vi "PCM_decode.vi"(8 "error in":errorcluster, 10 "inputData":dbl[](array[numeric]), 11 "Path In":path) -> (0 "error out":errorcluster, 2 "outData":dbl[](array[numeric]), 3 "Path Out":path)   [LabVIEW 2015]
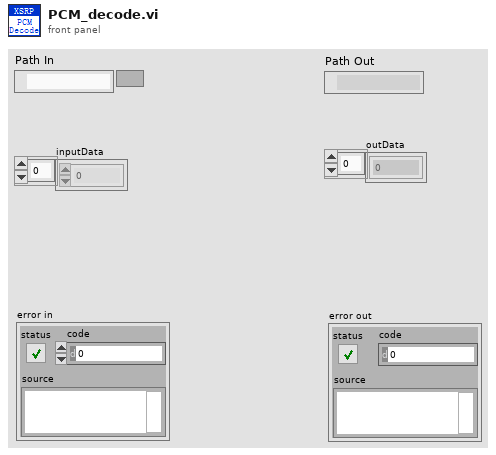
[diagram p1: front panel]
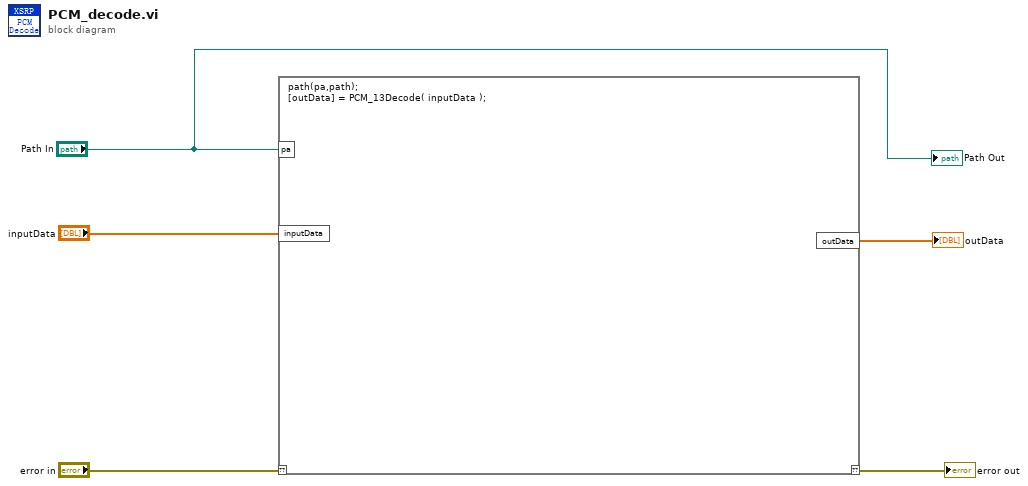
[diagram p0: block diagram]
diagram:
  n1 = script code="path(pa,path);\n[outData] = PCM_13Decode( inputData );"("??"="error in", "pa"="Path In", "inputData"="inputData") -> ("??"=→"error out":errorcluster, "outData"=→"outData":dbl[])
  "Path Out" <- "Path In"
